vi "Engine.vi"(7 "Action":T1, 8 "error in (no error)":errorcluster, 10 "skvc in":string[](array[string]), 11 "INI Path in":path) -> (0 "error out":errorcluster, 1 "Found?":bool, 2 "skvc out":string[](array[string]), 3 "INI Path out":path)   [LabVIEW 2018, in "Cfg.lvlib"]
uses:
  Cfg.lvlib
  Action.ctl
  <vilib>/ErrorRing/Error Ring.xnode
  <vilib>/Utility/error.llb/Error Cluster From Error Code.vi
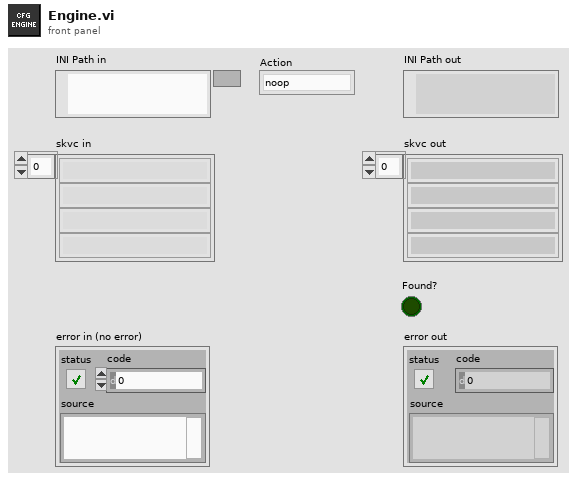
[diagram p1: front panel]
types:
  T1 = typedef "Cfg.lvlib/Action.ctl" = enum8{"noop", "new", "read_or_create", "read", "write", "remove", "keys", "sections", "remove_section", "import", "export", "get", "set", "pop", "add", "list", "list_sections", "pop_section"}
  T2 = cluster{"Paths":path[], "Files":cluster{"skvc":string[][]}[], "Modified":bool[], "LastMod":timestamp[], "PathIdx":i32, "Create":bool, "Found":bool, "skvc":string[]}
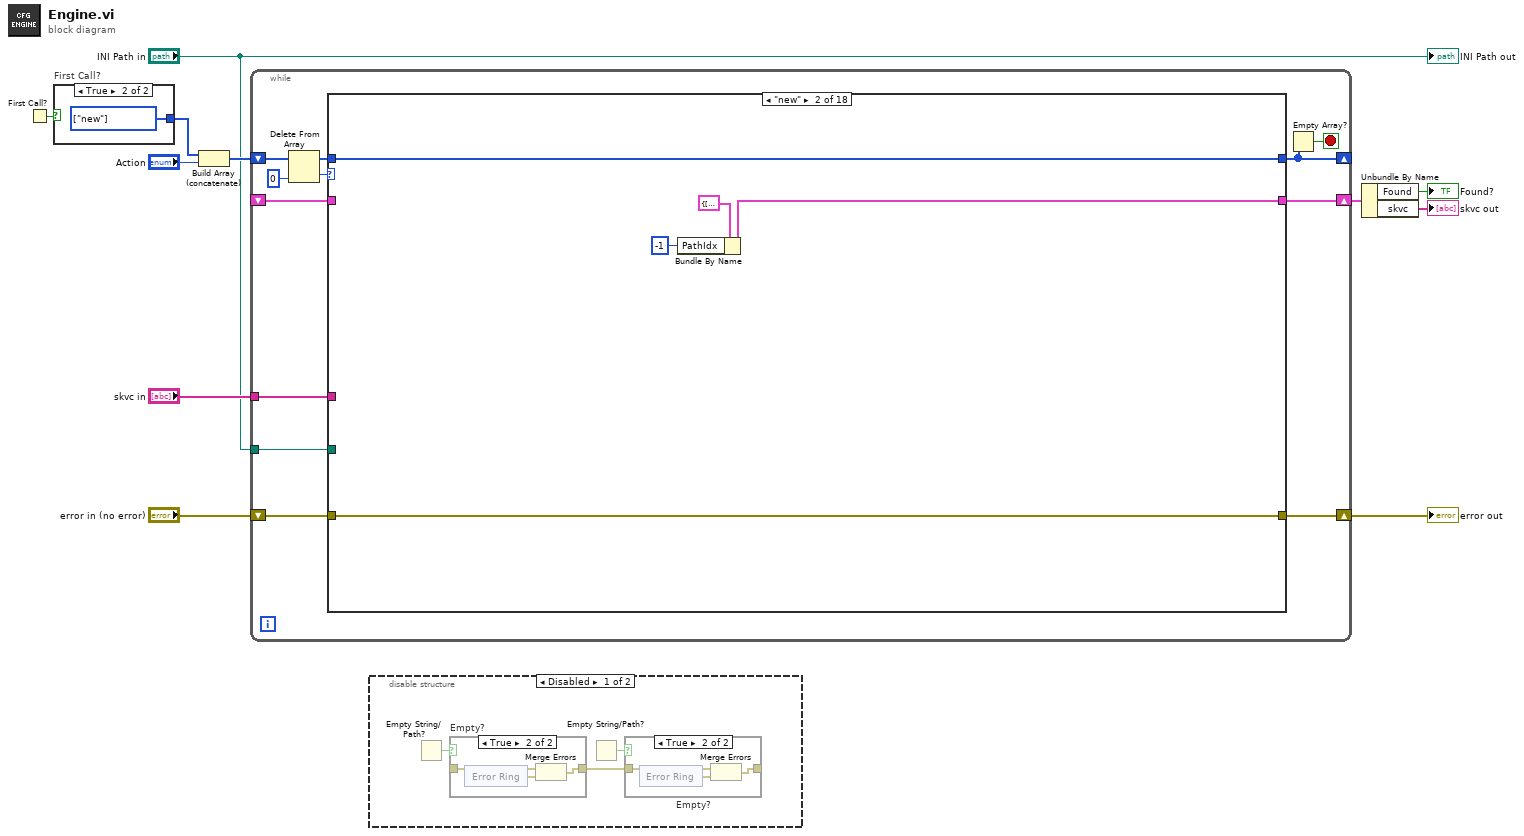
[diagram p0: block diagram]
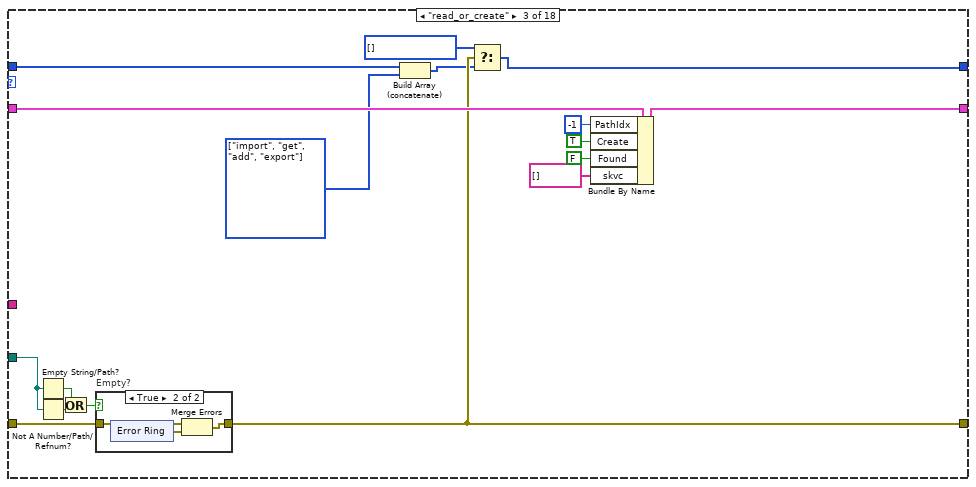
[diagram p6: hidden frame]
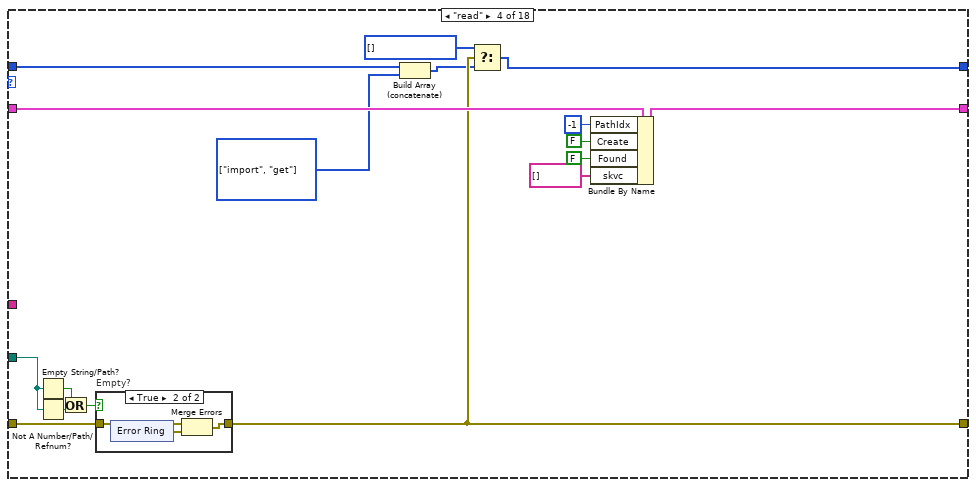
[diagram p8: hidden frame]
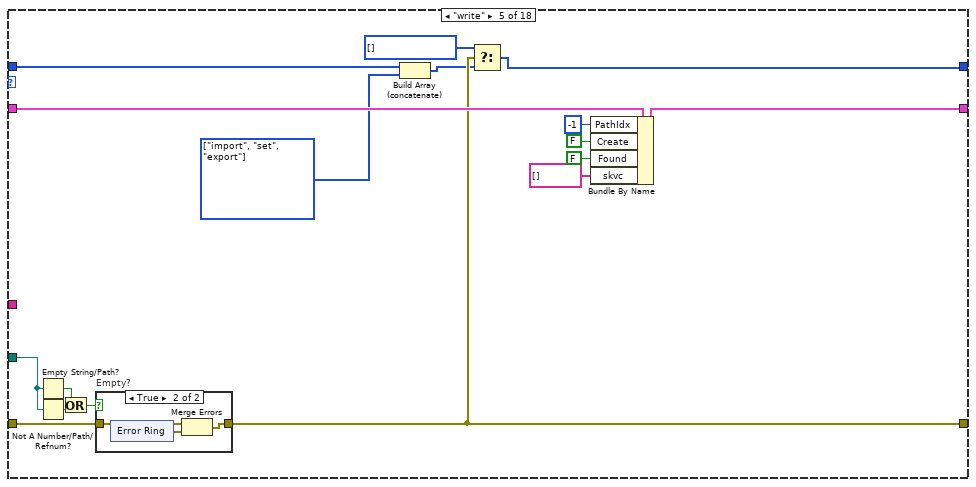
[diagram p10: hidden frame]
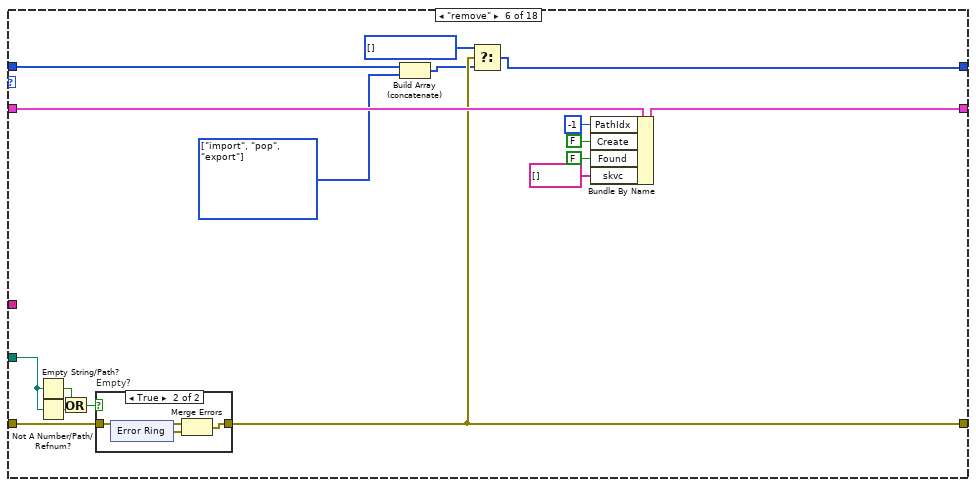
[diagram p12: hidden frame]
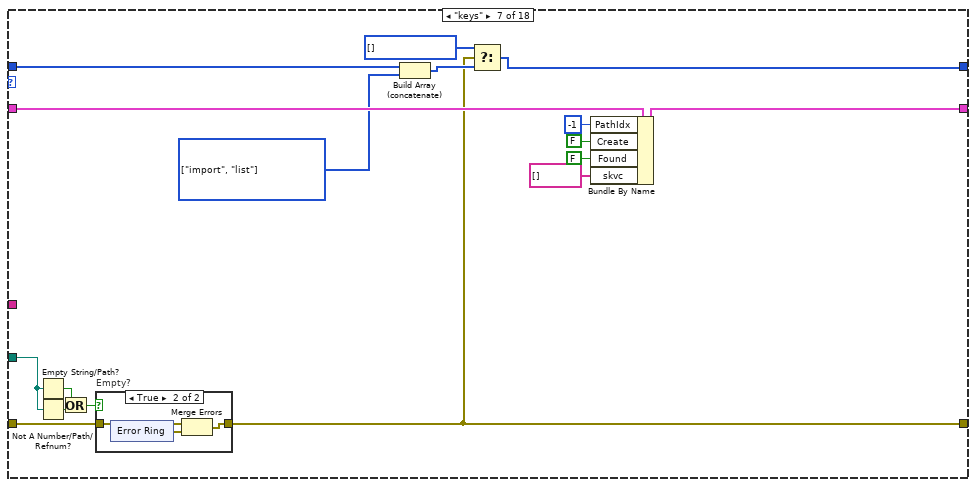
[diagram p14: hidden frame]
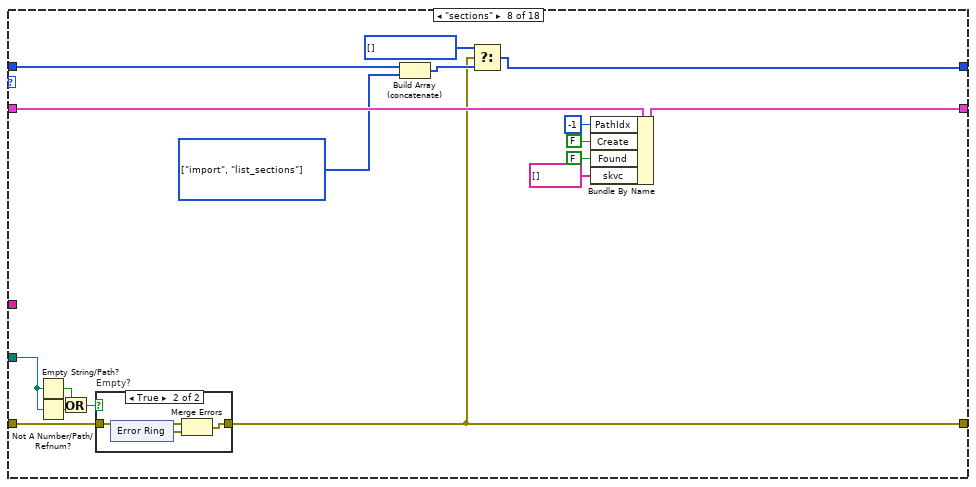
[diagram p16: hidden frame]
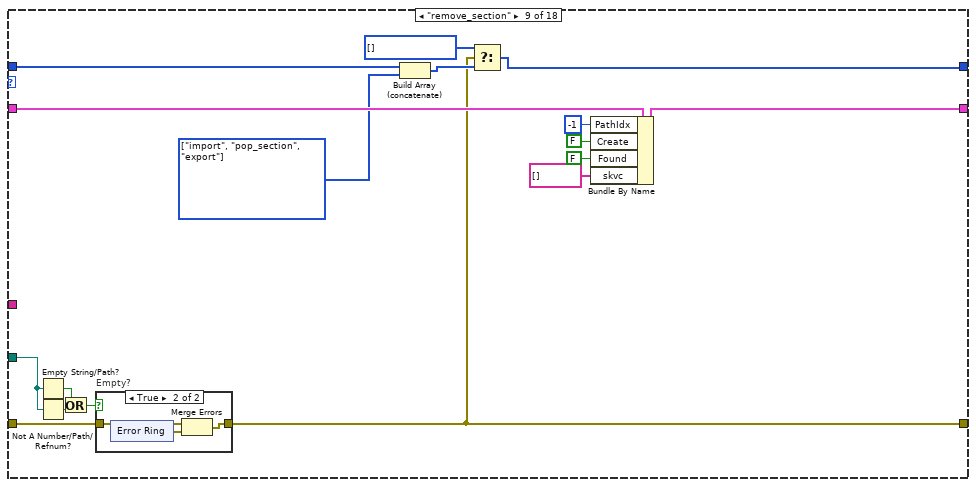
[diagram p18: hidden frame]
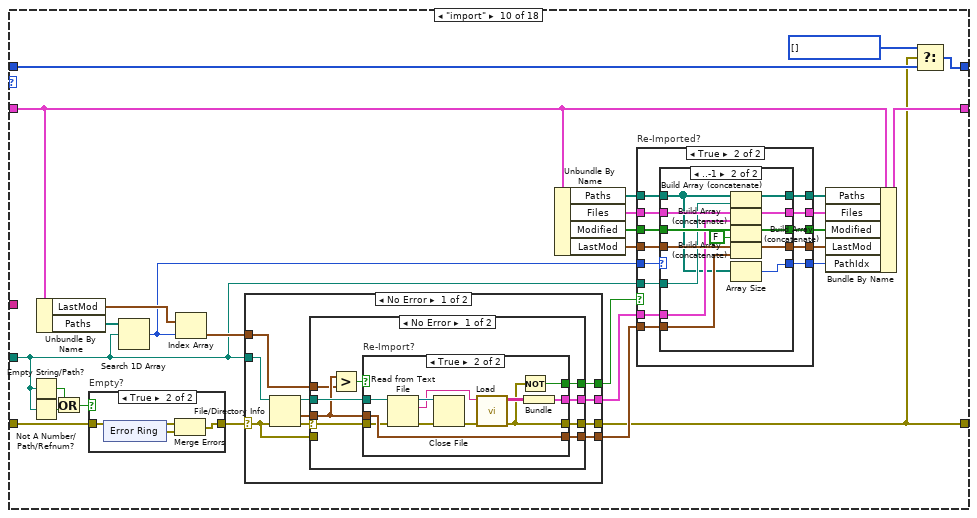
[diagram p20: hidden frame]
diagram:
  n1 = First Call?() -> (First Call?: T/F=w7:bool)
  n2 = case "First Call?" shown="True" w7 {
    tunnel: [_ w12] -> w6
    frame False {
    }
    frame True {
      w12 = T1[] [enum."new"] items=["noop", "new", "read_or_create", "read", "write", "remove", "keys", "sections", "remove_section", "import", "export", "get", "set", "pop", "add", "list", "list_sections", "pop_section"] ("appended array")
    }
  }
  n3 = Build Array (concatenate)(w6, "Action") -> (w8:T1[])
  n4 = while {
    shift-right: [w24] -> w11
    shift-left: "error in (no error)" -> [w23]
    shift-right: [w18] -> _
    shift-left: w8 -> [w22]
    shift-right: [w16] -> w3
    shift-left: _ -> [w15]
    tunnel: "INI Path in" -> [w14]
    tunnel: "skvc in" -> [w13]
    stop <- w17 stop-if-true
    n5 = Delete From Array(array=w22, index=0) -> (deleted portion=w19:T1, array with subset deleted=w21:T1[])  [unwired: 1 in]
    n6 = case shown="\"new\"" w19 {
      tunnel: [w27 w32 w41 w67 w93 w119 w137 w163 w189 w216 w339 w397 w428 w485 w529 w592 w615 w646] -> w24
      tunnel: w23 -> [w27 w32 w44 w70 w96 w122 w148 w174 w200 w241 w342 w397 w428 w485 w529 w592 w615 w646]
      tunnel: w21 -> [w26 w31 w49 w75 w101 w127 w153 w179 w205 w242 w350 w414 w431 w488 w538 w601 w622 w649]
      tunnel: [w26 w31 w42 w68 w94 w120 w146 w172 w198 w218 w350 w414 w431 w488 w538 w601 w622 w649] -> w18
      tunnel: [w25 w29 w37 w63 w89 w115 w142 w168 w194 w232 w331 w404 w429 w486 w536 w595 w616 w647] -> w16
      tunnel: w15 -> [w25 _ w48 w74 w100 w126 w152 w178 w204 w233 w336 w413 w430 w487 w537 w600 w621 w648]
      tunnel: w14 -> [_ _ w43 w69 w95 w121 w147 w173 w199 w221 w340 _ _ _ _ _ _ _]
      tunnel: w13 -> [_ _ _ _ _ _ _ _ _ _ _ w400 w426 w478 w534 w594 _ w639]
      frame "noop" {
      }
      frame "new" {
        n7 = Bundle By Name(cluster=T2 {"Paths"=[], "Files"=[], "Modified"=[], "LastMod"=[], "PathIdx"=0, "Create"=FALSE, "Found"=FALSE, "skvc"=[]} ("StateData"), "PathIdx"=-1) -> (w29:T2)
      }
      frame "read_or_create" {
        w38 = T1[] [enum."import", enum."get", enum."add", enum."export"] items=["noop", "new", "read_or_create", "read", "write", "remove", "keys", "sections", "remove_section", "import", "export", "get", "set", "pop", "add", "list", "list_sections", "pop_section"] ("element")
        w40 = T1[] [] items=["noop", "new", "read_or_create", "read", "write", "remove", "keys", "sections", "remove_section", "import", "export", "get", "set", "pop", "add", "list", "list_sections", "pop_section"] ("t")
        n8 = Empty String/Path?(string/path=w43) -> (empty?=w46:bool)
        n9 = Not A Number/Path/Refnum?(number/path/refnum=w43) -> (NaN/Path/Refnum?=w47:bool)
        n10 = Or(x=w46, y=w47) -> (x .or. y?=w45:bool)
        n11 = case "Empty?" shown="True" w45 {
          tunnel: w44 -> [w50 w53]
          tunnel: [w50 w52] -> w41
          frame False {
          }
          frame True {
            n12 = xnode "Error Ring"() -> ("error out"=w51:errorcluster)
            n13 = Merge Errors(w53, w51) -> (w52:errorcluster)
          }
        }
        n14 = Build Array (concatenate)(w49, w38) -> (w39:T1[])
        n15 = Select(t=w40, s=w41, f=w39) -> (s? t:f=w42:T1[])
        n16 = Bundle By Name(cluster=w48, "PathIdx"=-1, "Create"=TRUE, "Found"=FALSE, "skvc"=string[] []) -> (w37:T2)
      }
      frame "read" {
        w64 = T1[] [enum."import", enum."get"] items=["noop", "new", "read_or_create", "read", "write", "remove", "keys", "sections", "remove_section", "import", "export", "get", "set", "pop", "add", "list", "list_sections", "pop_section"] ("element")
        w66 = T1[] [] items=["noop", "new", "read_or_create", "read", "write", "remove", "keys", "sections", "remove_section", "import", "export", "get", "set", "pop", "add", "list", "list_sections", "pop_section"] ("t")
        n17 = Empty String/Path?(string/path=w69) -> (empty?=w72:bool)
        n18 = Not A Number/Path/Refnum?(number/path/refnum=w69) -> (NaN/Path/Refnum?=w73:bool)
        n19 = Or(x=w72, y=w73) -> (x .or. y?=w71:bool)
        n20 = case "Empty?" shown="True" w71 {
          tunnel: w70 -> [w76 w79]
          tunnel: [w76 w78] -> w67
          frame False {
          }
          frame True {
            n21 = xnode "Error Ring"() -> ("error out"=w77:errorcluster)
            n22 = Merge Errors(w79, w77) -> (w78:errorcluster)
          }
        }
        n23 = Build Array (concatenate)(w75, w64) -> (w65:T1[])
        n24 = Select(t=w66, s=w67, f=w65) -> (s? t:f=w68:T1[])
        n25 = Bundle By Name(cluster=w74, "PathIdx"=-1, "Create"=FALSE, "Found"=FALSE, "skvc"=string[] []) -> (w63:T2)
      }
      frame "write" {
        w90 = T1[] [enum."import", enum."set", enum."export"] items=["noop", "new", "read_or_create", "read", "write", "remove", "keys", "sections", "remove_section", "import", "export", "get", "set", "pop", "add", "list", "list_sections", "pop_section"] ("element")
        w92 = T1[] [] items=["noop", "new", "read_or_create", "read", "write", "remove", "keys", "sections", "remove_section", "import", "export", "get", "set", "pop", "add", "list", "list_sections", "pop_section"] ("t")
        n26 = Empty String/Path?(string/path=w95) -> (empty?=w98:bool)
        n27 = Not A Number/Path/Refnum?(number/path/refnum=w95) -> (NaN/Path/Refnum?=w99:bool)
        n28 = Or(x=w98, y=w99) -> (x .or. y?=w97:bool)
        n29 = case "Empty?" shown="True" w97 {
          tunnel: w96 -> [w102 w105]
          tunnel: [w102 w104] -> w93
          frame False {
          }
          frame True {
            n30 = xnode "Error Ring"() -> ("error out"=w103:errorcluster)
            n31 = Merge Errors(w105, w103) -> (w104:errorcluster)
          }
        }
        n32 = Build Array (concatenate)(w101, w90) -> (w91:T1[])
        n33 = Select(t=w92, s=w93, f=w91) -> (s? t:f=w94:T1[])
        n34 = Bundle By Name(cluster=w100, "PathIdx"=-1, "Create"=FALSE, "Found"=FALSE, "skvc"=string[] []) -> (w89:T2)
      }
      frame "remove" {
        w116 = T1[] [enum."import", enum."pop", enum."export"] items=["noop", "new", "read_or_create", "read", "write", "remove", "keys", "sections", "remove_section", "import", "export", "get", "set", "pop", "add", "list", "list_sections", "pop_section"] ("element")
        w118 = T1[] [] items=["noop", "new", "read_or_create", "read", "write", "remove", "keys", "sections", "remove_section", "import", "export", "get", "set", "pop", "add", "list", "list_sections", "pop_section"] ("t")
        n35 = Empty String/Path?(string/path=w121) -> (empty?=w124:bool)
        n36 = Not A Number/Path/Refnum?(number/path/refnum=w121) -> (NaN/Path/Refnum?=w125:bool)
        n37 = Or(x=w124, y=w125) -> (x .or. y?=w123:bool)
        n38 = case "Empty?" shown="True" w123 {
          tunnel: w122 -> [w128 w131]
          tunnel: [w128 w130] -> w119
          frame False {
          }
          frame True {
            n39 = xnode "Error Ring"() -> ("error out"=w129:errorcluster)
            n40 = Merge Errors(w131, w129) -> (w130:errorcluster)
          }
        }
        n41 = Build Array (concatenate)(w127, w116) -> (w117:T1[])
        n42 = Select(t=w118, s=w119, f=w117) -> (s? t:f=w120:T1[])
        n43 = Bundle By Name(cluster=w126, "PathIdx"=-1, "Create"=FALSE, "Found"=FALSE, "skvc"=string[] []) -> (w115:T2)
      }
      frame "keys" {
        w143 = T1[] [enum."import", enum."list"] items=["noop", "new", "read_or_create", "read", "write", "remove", "keys", "sections", "remove_section", "import", "export", "get", "set", "pop", "add", "list", "list_sections", "pop_section"] ("element")
        w145 = T1[] [] items=["noop", "new", "read_or_create", "read", "write", "remove", "keys", "sections", "remove_section", "import", "export", "get", "set", "pop", "add", "list", "list_sections", "pop_section"] ("t")
        n44 = Empty String/Path?(string/path=w147) -> (empty?=w150:bool)
        n45 = Not A Number/Path/Refnum?(number/path/refnum=w147) -> (NaN/Path/Refnum?=w151:bool)
        n46 = Or(x=w150, y=w151) -> (x .or. y?=w149:bool)
        n47 = case "Empty?" shown="True" w149 {
          tunnel: w148 -> [w154 w157]
          tunnel: [w154 w156] -> w137
          frame False {
          }
          frame True {
            n48 = xnode "Error Ring"() -> ("error out"=w155:errorcluster)
            n49 = Merge Errors(w157, w155) -> (w156:errorcluster)
          }
        }
        n50 = Build Array (concatenate)(w153, w143) -> (w144:T1[])
        n51 = Select(t=w145, s=w137, f=w144) -> (s? t:f=w146:T1[])
        n52 = Bundle By Name(cluster=w152, "PathIdx"=-1, "Create"=FALSE, "Found"=FALSE, "skvc"=string[] []) -> (w142:T2)
      }
      frame "sections" {
        w169 = T1[] [enum."import", enum."list_sections"] items=["noop", "new", "read_or_create", "read", "write", "remove", "keys", "sections", "remove_section", "import", "export", "get", "set", "pop", "add", "list", "list_sections", "pop_section"] ("element")
        w171 = T1[] [] items=["noop", "new", "read_or_create", "read", "write", "remove", "keys", "sections", "remove_section", "import", "export", "get", "set", "pop", "add", "list", "list_sections", "pop_section"] ("t")
        n53 = Empty String/Path?(string/path=w173) -> (empty?=w176:bool)
        n54 = Not A Number/Path/Refnum?(number/path/refnum=w173) -> (NaN/Path/Refnum?=w177:bool)
        n55 = Or(x=w176, y=w177) -> (x .or. y?=w175:bool)
        n56 = case "Empty?" shown="True" w175 {
          tunnel: w174 -> [w180 w183]
          tunnel: [w180 w182] -> w163
          frame False {
          }
          frame True {
            n57 = xnode "Error Ring"() -> ("error out"=w181:errorcluster)
            n58 = Merge Errors(w183, w181) -> (w182:errorcluster)
          }
        }
        n59 = Build Array (concatenate)(w179, w169) -> (w170:T1[])
        n60 = Select(t=w171, s=w163, f=w170) -> (s? t:f=w172:T1[])
        n61 = Bundle By Name(cluster=w178, "PathIdx"=-1, "Create"=FALSE, "Found"=FALSE, "skvc"=string[] []) -> (w168:T2)
      }
      frame "remove_section" {
        w195 = T1[] [enum."import", enum."pop_section", enum."export"] items=["noop", "new", "read_or_create", "read", "write", "remove", "keys", "sections", "remove_section", "import", "export", "get", "set", "pop", "add", "list", "list_sections", "pop_section"] ("element")
        w197 = T1[] [] items=["noop", "new", "read_or_create", "read", "write", "remove", "keys", "sections", "remove_section", "import", "export", "get", "set", "pop", "add", "list", "list_sections", "pop_section"] ("t")
        n62 = Empty String/Path?(string/path=w199) -> (empty?=w202:bool)
        n63 = Not A Number/Path/Refnum?(number/path/refnum=w199) -> (NaN/Path/Refnum?=w203:bool)
        n64 = Or(x=w202, y=w203) -> (x .or. y?=w201:bool)
        n65 = case "Empty?" shown="True" w201 {
          tunnel: w200 -> [w206 w209]
          tunnel: [w206 w208] -> w189
          frame False {
          }
          frame True {
            n66 = xnode "Error Ring"() -> ("error out"=w207:errorcluster)
            n67 = Merge Errors(w209, w207) -> (w208:errorcluster)
          }
        }
        n68 = Build Array (concatenate)(w205, w195) -> (w196:T1[])
        n69 = Select(t=w197, s=w189, f=w196) -> (s? t:f=w198:T1[])
        n70 = Bundle By Name(cluster=w204, "PathIdx"=-1, "Create"=FALSE, "Found"=FALSE, "skvc"=string[] []) -> (w194:T2)
      }
      frame "import" {
        w217 = T1[] [] items=["noop", "new", "read_or_create", "read", "write", "remove", "keys", "sections", "remove_section", "import", "export", "get", "set", "pop", "add", "list", "list_sections", "pop_section"] ("t")
        n71 = Empty String/Path?(string/path=w221) -> (empty?=w237:bool)
        n72 = Not A Number/Path/Refnum?(number/path/refnum=w221) -> (NaN/Path/Refnum?=w238:bool)
        n73 = Unbundle By Name(w233) -> ("LastMod"=w240:timestamp[], "Paths"=w234:path[])
        n74 = Or(x=w237, y=w238) -> (x .or. y?=w236:bool)
        n75 = case "Empty?" shown="True" w236 {
          tunnel: w241 -> [w319 w322]
          tunnel: [w319 w321] -> w235
          frame False {
          }
          frame True {
            n76 = xnode "Error Ring"() -> ("error out"=w320:errorcluster)
            n77 = Merge Errors(w322, w320) -> (w321:errorcluster)
          }
        }
        n78 = Search 1D Array(1D array=w234, element=w221) -> (index of element=w219:i32)  [unwired: 1 in]
        n79 = Index Array(array=w240, index=w219) -> (element=w239:timestamp)
        n80 = case shown="No Error" w235 {
          selector: w235 -> [w288 w318]
          tunnel: [w294 w318] -> w216
          tunnel: w239 -> [w290 _]
          tunnel: w221 -> [w289 _]
          tunnel: [w287 _] -> w222
          tunnel: [w286 _] -> w220
          tunnel: [w285 _] -> w223
          frame No Error {
            n81 = File/Directory Info(path=w289, error in=w288) -> (path out=w292:path, last mod=w291:timestamp, error out=w293:errorcluster)  [unwired: 4 out]
            n82 = case shown="No Error" w293 {
              selector: w293 -> [w296 _]
              tunnel: [w297 w317] -> w294
              tunnel: w292 -> [w303 _]
              tunnel: w291 -> [w301 _]
              tunnel: w290 -> [w298 _]
              tunnel: w288 -> [_ w317]
              tunnel: [w300 _] -> w287
              tunnel: [w299 _] -> w286
              tunnel: [w295 TRUE] -> w285
              frame No Error {
                n83 = Greater?(x=w301, y=w298) -> (0:w302:bool)
                n84 = case "Re-Import?" shown="True" w302 {
                  tunnel: w303 -> [_ w315]
                  tunnel: w301 -> [_ w309]
                  tunnel: [_ w305] -> w300
                  tunnel: [_ w309] -> w299
                  tunnel: [w304 w307] -> w297
                  tunnel: w296 -> [w304 w308]
                  tunnel: [_ w306] -> w295
                  frame False {
                  }
                  frame True {
                    n85 = Read from Text File(file (use dialog)=w315, error in=w308) -> (refnum out=w313:refnum<file>, text=w311:string, error out=w314:errorcluster)  [unwired: 2 in, 1 out]
                    n86 = Close File(refnum=w313, error in=w314) -> (error out=w312:errorcluster)  [unwired: 1 out]
                    n87 = call "Load.vi"("error in (no error)"=w312, "Text"=w311) -> ("error out"=w307:errorcluster, "skvc"=w310:string[][])  [unwired: 8 in]
                    n88 = Not(x=w307) -> (.not. x?=w306:bool)
                    n89 = Bundle("skvc"=w310) -> (w305:cluster{"skvc":string[][]})  [unwired: 1 in]
                  }
                }
              }
              frame Error {
                # "File does not exist"
              }
            }
          }
          frame Error {
          }
        }
        n90 = Unbundle By Name(w233) -> ("Paths"=w231:path[], "Files"=w230:cluster{"skvc":string[][]}[], "Modified"=w229:bool[], "LastMod"=w228:timestamp[])
        n91 = case "Re-Imported?" shown="True" w223 {
          tunnel: w231 -> [w247 w260]
          tunnel: w230 -> [w246 w259]
          tunnel: w229 -> [w245 w258]
          tunnel: w228 -> [w244 w257]
          tunnel: [w244 w256] -> w227
          tunnel: [w245 w255] -> w226
          tunnel: [w246 w254] -> w225
          tunnel: [w247 w253] -> w224
          tunnel: w222 -> [_ w252]
          tunnel: w221 -> [_ w251]
          tunnel: w220 -> [_ w250]
          tunnel: w219 -> [w243 w249]
          tunnel: [w243 w248] -> w215
          frame False {
          }
          frame True {
            n92 = case shown="..-1" w249 {
              selector: w249 -> [w262 _]
              tunnel: w260 -> [w271 w273]
              tunnel: w259 -> [w270 w284]
              tunnel: w258 -> [w264 w283]
              tunnel: w257 -> [w266 w282]
              tunnel: [w265 w281] -> w256
              tunnel: [w263 w280] -> w255
              tunnel: [w269 w279] -> w254
              tunnel: [w271 w278] -> w253
              tunnel: w252 -> [w268 w277]
              tunnel: w251 -> [_ w276]
              tunnel: w250 -> [w267 w274]
              tunnel: [w262 w272] -> w248
              frame 0.. {
                n93 = Replace Array Subset(array=w270, new element=w268, index=w262) -> (w269:cluster{"skvc":string[][]}[])
                n94 = Replace Array Subset(array=w264, new element=FALSE ("new element/subarray"), index=w262) -> (w263:bool[])
                n95 = Replace Array Subset(array=w266, new element=w267, index=w262) -> (w265:timestamp[])
              }
              frame ..-1 {
                n96 = Build Array (concatenate)(w273, w276) -> (w278:path[])
                n97 = Build Array (concatenate)(w284, w277) -> (w279:cluster{"skvc":string[][]}[])
                n98 = Build Array (concatenate)(w283, FALSE ("Boolean")) -> (w280:bool[])
                n99 = Build Array (concatenate)(w282, w274) -> (w281:timestamp[])
                n100 = Array Size(array=w273) -> (size(s)=w272:i32)
              }
            }
          }
        }
        n101 = Bundle By Name(cluster=w233, "Paths"=w224, "Files"=w225, "Modified"=w226, "LastMod"=w227, "PathIdx"=w215) -> (w232:T2)
        n102 = Select(t=w217, s=w216, f=w242) -> (s? t:f=w218:T1[])
      }
      frame "export" {
        n103 = Empty String/Path?(string/path=w340) -> (empty?=w345:bool)
        n104 = Not A Number/Path/Refnum?(number/path/refnum=w340) -> (NaN/Path/Refnum?=w346:bool)
        n105 = Unbundle By Name(w336) -> ("Files"=w347:cluster{"skvc":string[][]}[], "Modified"=w348:bool[], "Paths"=w349:path[])
        n106 = Or(x=w345, y=w346) -> (x .or. y?=w344:bool)
        n107 = case "Empty?" shown="True" w344 {
          tunnel: w342 -> [w387 w390]
          tunnel: [w387 w389] -> w343
          frame False {
          }
          frame True {
            n108 = xnode "Error Ring"() -> ("error out"=w388:errorcluster)
            n109 = Merge Errors(w390, w388) -> (w389:errorcluster)
          }
        }
        n110 = Search 1D Array(1D array=w349, element=w340) -> (index of element=w332:i32)  [unwired: 1 in]
        n111 = Index Array(array=w347, index=w332) -> (element=w341:cluster{"skvc":string[][]})
        n112 = Index Array(array=w348, index=w332) -> (element=w338:bool)
        n113 = Unbundle By Name(w341) -> ("skvc"=w337:string[][])
        n114 = case "Modified?" shown="True" w338 {
          tunnel: w343 -> [w360 w366]
          tunnel: w340 -> [_ w365]
          tunnel: [w360 w364] -> w339
          tunnel: w337 -> [_ w362]
          tunnel: [_ w363] -> w334
          tunnel: [_ w361] -> w328
          frame False {
          }
          frame True {
            n115 = case shown="No Error" w366 {
              selector: w366 -> [w382 w386]
              tunnel: w365 -> [w377 _]
              tunnel: [w372 w386] -> w364
              tunnel: [w373 _] -> w363
              tunnel: w362 -> [w367 _]
              tunnel: [w371 _] -> w361
              frame No Error {
                n116 = Strip Path(path=w377) -> (stripped path=w380:path)  [unwired: 1 out]
                n117 = File/Directory Info(path=w380, error in=w382) -> (path out=w379:path, error out=w381:errorcluster)  [unwired: 5 out]
                n118 = case shown="Error .." w381 {
                  selector: w381 -> [w383 _]
                  tunnel: [w383 w385] -> w370
                  tunnel: w379 -> [_ w384]
                  frame No Error {
                  }
                  frame Error {
                    n119 = Create Folder(path (use dialog)=w384) -> (error out=w385:errorcluster)  [unwired: 2 in, 2 out]
                  }
                }
                n120 = call "Dump.vi"("error in (no error)"=w370, "skvc"=w367) -> ("error out"=w369:errorcluster, "Text"=w368:string)  [unwired: 8 in]
                n121 = Write to Text File(file (use dialog)=w377, text=w368, error in=w369) -> (refnum out=w375:refnum<file>, error out=w378:errorcluster)  [unwired: 1 in, 1 out]
                n122 = Close File(refnum=w375, error in=w378) -> (path=w374:path, error out=w376:errorcluster)
                n123 = File/Directory Info(path=w374, error in=w376) -> (last mod=w373:timestamp, error out=w372:errorcluster)  [unwired: 5 out]
                n124 = Not(x=w372) -> (.not. x?=w371:bool)
              }
              frame Error {
              }
            }
          }
        }
        n125 = Unbundle By Name(w336) -> ("Modified"=w333:bool[], "LastMod"=w335:timestamp[])
        n126 = case "Written?" shown="True" w328 {
          tunnel: w335 -> [w351 w359]
          tunnel: w334 -> [_ w358]
          tunnel: w333 -> [w352 w357]
          tunnel: w332 -> [_ w355]
          tunnel: [w352 w354] -> w330
          tunnel: [w351 w353] -> w329
          frame False {
          }
          frame True {
            n127 = Replace Array Subset(array=w357, new element=FALSE ("new element/subarray"), index=w355) -> (w354:bool[])
            n128 = Replace Array Subset(array=w359, new element=w358, index=w355) -> (w353:timestamp[])
          }
        }
        n129 = Bundle By Name(cluster=w336, "Modified"=w330, "LastMod"=w329) -> (w331:T2)
      }
      frame "get" {
        n130 = Unbundle By Name(w413) -> ("Files"=w412:cluster{"skvc":string[][]}[], "PathIdx"=w411:i32)
        n131 = Index Array(array=w412, index=w411) -> (element=w410:cluster{"skvc":string[][]})
        n132 = Unbundle By Name(w410) -> ("skvc"=w405:string[][])
        n133 = for {
          tunnel: w405 -> [w420] mode=indexing
          tunnel: [w417] -> w409 mode=indexing
          n134 = Index Array(array=w420) -> (element #1=w419:string, element #2=w418:string)  [unwired: 2 in]
          n135 = To Upper Case(1:w419) -> (0:w415:string)
          n136 = To Upper Case(1:w418) -> (0:w416:string)
          n137 = Bundle(w415, w416) -> (w417:cluster{string, string})  [unwired: 1 in]
        }
        n138 = Index Array(array=w400) -> (element #1=w399:string, element #2=w398:string)  [unwired: 2 in]
        n139 = To Upper Case(1:w399) -> (0:w408:string)
        n140 = To Upper Case(1:w398) -> (0:w407:string)
        n141 = Bundle(w408, w407) -> (w406:cluster{string, string})  [unwired: 1 in]
        n142 = Search 1D Array(1D array=w409, element=w406) -> (index of element=w403:i32)  [unwired: 1 in]
        n143 = Greater Or Equal To 0?(x=w403) -> (x >= 0?=w396:bool)
        n144 = Index Array(array=w405, index (row)=w403) -> (element=w402:string[])  [unwired: 1 in]
        n145 = Select(t=w402, s=w396, f=w400) -> (s? t:f=w401:string[])
        n146 = Bundle By Name(cluster=w413, "skvc"=w401, "Found"=w396) -> (w404:T2)
      }
      frame "set" {
        n147 = Unbundle By Name(w430) -> ("Modified"=w423:bool[], "Files"=w427:cluster{"skvc":string[][]}[], "PathIdx"=w424:i32)
        n148 = in-place {
          in-place-border: w426 -> [w437]
          in-place-border: [w432] -> w421
          n149 = in-place-array #1(w423, w424) -> (w434:bool)
          n150 = in-place-array #2(w427, w424) -> (w436:cluster{"skvc":string[][]})
          n151 = in-place {
            in-place-border: w437 -> [w441]
            in-place-border: w434 -> [w440]
            in-place-border: [w439] -> w433
            in-place-border: [w438] -> w432
            n152 = in-place-cluster #3(w436) -> ("skvc"=w443:string[][])
            n153 = for {
              tunnel: w443 -> [w476] mode=indexing
              tunnel: [w473] -> w450 mode=indexing
              n154 = Index Array(array=w476) -> (element #1=w475:string, element #2=w474:string)  [unwired: 2 in]
              n155 = To Upper Case(1:w475) -> (0:w471:string)
              n156 = To Upper Case(1:w474) -> (0:w472:string)
              n157 = Bundle(w471, w472) -> (w473:cluster{string, string})  [unwired: 1 in]
            }
            n158 = Index Array(array=w441) -> (element #1=w446:string, element #2=w445:string)  [unwired: 2 in]
            n159 = To Upper Case(1:w446) -> (0:w449:string)
            n160 = To Upper Case(1:w445) -> (0:w448:string)
            n161 = Bundle(w449, w448) -> (w447:cluster{string, string})  [unwired: 1 in]
            n162 = Search 1D Array(1D array=w450, element=w447) -> (index of element=w444:i32)  [unwired: 1 in]
            n163 = case shown="0.." w444 {
              selector: w444 -> [w455 _]
              tunnel: w443 -> [w458 w470]
              tunnel: [w456 w469] -> w442
              tunnel: w441 -> [w454 w468]
              tunnel: w440 -> [w453 _]
              tunnel: [w452 w467] -> w439
              tunnel: [w451 w466] -> w438
              frame 0.. {
                w451 = TRUE  # Found?
                n164 = in-place {
                  in-place-border: w454 -> [w465]
                  in-place-border: w453 -> [w462]
                  in-place-border: [w460] -> w452
                  n165 = in-place-array #4(w458, w455, 2) -> (w463:string)
                  n166 = Index Array(array=w465, index=2) -> (element=w459:string)
                  n167 = Not Equal?(x=w463, y=w459) -> (x != y?=w461:bool)
                  n168 = Or(x=w462, y=w461) -> (x .or. y?=w460:bool)
                  n169 = in-place-array #4(w459) -> (w456:string[][])  [unwired: 2 out]
                }
              }
              frame ..-1 {
                w466 = FALSE  # Found?
                w467 = TRUE  # Modified?
                n170 = Build Array (concatenate)(w470, w468) -> (w469:string[][])
              }
            }
            n171 = in-place-cluster #3("skvc"=w442) -> (w435:cluster{"skvc":string[][]})
          }
          n172 = in-place-array #1(w433) -> (w422:bool[])  [unwired: 1 out]
          n173 = in-place-array #2(w435) -> (w425:cluster{"skvc":string[][]}[])  [unwired: 1 out]
        }
        n174 = Bundle By Name(cluster=w430, "Modified"=w422, "Files"=w425, "Found"=w421, "skvc"=w426) -> (w429:T2)
      }
      frame "pop" {
        n175 = Unbundle By Name(w487) -> ("Modified"=w481:bool[], "Files"=w484:cluster{"skvc":string[][]}[], "PathIdx"=w482:i32)
        n176 = in-place {
          in-place-border: w478 -> [w495]
          in-place-border: [w490] -> w479
          in-place-border: [w489] -> w477
          n177 = in-place-array #5(w481, w482) -> (w492:bool)
          n178 = in-place-array #6(w484, w482) -> (w494:cluster{"skvc":string[][]})
          n179 = in-place {
            in-place-border: w495 -> [w497]
            in-place-border: w492 -> [w501]
            in-place-border: [w500] -> w491
            in-place-border: [w499] -> w490
            in-place-border: [w496] -> w489
            n180 = in-place-cluster #7(w494) -> ("skvc"=w502:string[][])
            n181 = for {
              tunnel: w502 -> [w525] mode=indexing
              tunnel: [w522] -> w509 mode=indexing
              n182 = Index Array(array=w525) -> (element #1=w524:string, element #2=w523:string)  [unwired: 2 in]
              n183 = To Upper Case(1:w524) -> (0:w520:string)
              n184 = To Upper Case(1:w523) -> (0:w521:string)
              n185 = Bundle(w520, w521) -> (w522:cluster{string, string})  [unwired: 1 in]
            }
            n186 = Index Array(array=w497) -> (element #1=w505:string, element #2=w504:string)  [unwired: 2 in]
            n187 = To Upper Case(1:w505) -> (0:w508:string)
            n188 = To Upper Case(1:w504) -> (0:w507:string)
            n189 = Bundle(w508, w507) -> (w506:cluster{string, string})  [unwired: 1 in]
            n190 = Search 1D Array(1D array=w509, element=w506) -> (index of element=w503:i32)  [unwired: 1 in]
            n191 = case shown="0.." w503 {
              selector: w503 -> [w513 _]
              tunnel: w502 -> [w514 w518]
              tunnel: w501 -> [_ w517]
              tunnel: [w511 w517] -> w500
              tunnel: [w515 w519] -> w499
              tunnel: [w512 w518] -> w498
              tunnel: w497 -> [_ w516]
              tunnel: [w510 w516] -> w496
              frame 0.. {
                w511 = TRUE  # Modified?
                w515 = TRUE  # Found?
                n192 = Delete From Array(array=w514, index (row)=w513) -> (deleted portion=w510:string[], array with subset deleted=w512:string[][])  [unwired: 2 in]
              }
              frame ..-1 {
                w519 = FALSE  # Found?
              }
            }
            n193 = in-place-cluster #7("skvc"=w498) -> (w493:cluster{"skvc":string[][]})
          }
          n194 = in-place-array #5(w491) -> (w480:bool[])  [unwired: 1 out]
          n195 = in-place-array #6(w493) -> (w483:cluster{"skvc":string[][]}[])  [unwired: 1 out]
        }
        n196 = Bundle By Name(cluster=w487, "Modified"=w480, "Files"=w483, "Found"=w479, "skvc"=w477) -> (w486:T2)
      }
      frame "add" {
        n197 = Unbundle By Name(w537) -> ("Create"=w528:bool, "Found"=w527:bool, "Modified"=w531:bool[], "Files"=w535:cluster{"skvc":string[][]}[], "PathIdx"=w532:i32)
        n198 = Compound Arithmetic op=AND(w528, invert w527) -> (w526:bool)
        n199 = case "Create Key?" shown="True" w526 {
          tunnel: w535 -> [w539 w546]
          tunnel: w534 -> [_ w545]
          tunnel: [w539 w544] -> w533
          tunnel: w532 -> [_ w543]
          tunnel: w531 -> [w540 w542]
          tunnel: [w540 w541] -> w530
          frame False {
          }
          frame True {
            n200 = in-place {
              in-place-border: w545 -> [w551]
              n201 = in-place-array #8(w542, w543) -> (w548:bool)
              n202 = in-place-array #9(w546, w543) -> (w550:cluster{"skvc":string[][]})
              n203 = in-place {
                in-place-border: w551 -> [w554]
                in-place-border: w548 -> [w553]
                in-place-border: [w552] -> w547
                n204 = in-place-cluster #10(w550) -> ("skvc"=w556:string[][])
                n205 = for {
                  tunnel: w556 -> [w587] mode=indexing
                  tunnel: [w584] -> w563 mode=indexing
                  n206 = Index Array(array=w587) -> (element #1=w586:string, element #2=w585:string)  [unwired: 2 in]
                  n207 = To Upper Case(1:w586) -> (0:w582:string)
                  n208 = To Upper Case(1:w585) -> (0:w583:string)
                  n209 = Bundle(w582, w583) -> (w584:cluster{string, string})  [unwired: 1 in]
                }
                n210 = Index Array(array=w554) -> (element #1=w559:string, element #2=w558:string)  [unwired: 2 in]
                n211 = To Upper Case(1:w559) -> (0:w562:string)
                n212 = To Upper Case(1:w558) -> (0:w561:string)
                n213 = Bundle(w562, w561) -> (w560:cluster{string, string})  [unwired: 1 in]
                n214 = Search 1D Array(1D array=w563, element=w560) -> (index of element=w557:i32)  [unwired: 1 in]
                n215 = case shown="0.." w557 {
                  selector: w557 -> [w567 _]
                  tunnel: w556 -> [w570 w581]
                  tunnel: [w568 w580] -> w555
                  tunnel: w554 -> [w566 w579]
                  tunnel: w553 -> [w565 _]
                  tunnel: [w564 w578] -> w552
                  frame 0.. {
                    n216 = in-place {
                      in-place-border: w566 -> [w577]
                      in-place-border: w565 -> [w574]
                      in-place-border: [w572] -> w564
                      n217 = in-place-array #11(w570, w567, 2) -> (w575:string)
                      n218 = Index Array(array=w577, index=2) -> (element=w571:string)
                      n219 = Not Equal?(x=w575, y=w571) -> (x != y?=w573:bool)
                      n220 = Or(x=w574, y=w573) -> (x .or. y?=w572:bool)
                      n221 = in-place-array #11(w571) -> (w568:string[][])  [unwired: 2 out]
                    }
                  }
                  frame ..-1 {
                    w578 = TRUE  # Modified?
                    n222 = Build Array (concatenate)(w581, w579) -> (w580:string[][])
                  }
                }
                n223 = in-place-cluster #10("skvc"=w555) -> (w549:cluster{"skvc":string[][]})
              }
              n224 = in-place-array #8(w547) -> (w541:bool[])  [unwired: 1 out]
              n225 = in-place-array #9(w549) -> (w544:cluster{"skvc":string[][]}[])  [unwired: 1 out]
            }
          }
        }
        n226 = Bundle By Name(cluster=w537, "Modified"=w530, "Files"=w533) -> (w536:T2)
      }
      frame "list" {
        n227 = Unbundle By Name(w600) -> ("Files"=w599:cluster{"skvc":string[][]}[], "PathIdx"=w598:i32)
        n228 = Index Array(array=w594) -> (element=w593:string)  [unwired: 1 in]
        n229 = Index Array(array=w599, index=w598) -> (element=w597:cluster{"skvc":string[][]})
        n230 = To Upper Case(1:w593) -> (0:w591:string)
        n231 = Unbundle By Name(w597) -> ("skvc"=w596:string[][])
        n232 = for {
          tunnel: w596 -> [w611] mode=indexing
          tunnel: [w607] -> w590 mode=indexing if=w605
          tunnel: w591 -> [w608]
          shift-right: [w603] -> w588
          shift-left: FALSE -> [w602]
          n233 = Index Array(array=w611) -> (element #1=w610:string, element #2=w607:string)  [unwired: 2 in]
          n234 = To Upper Case(1:w610) -> (0:w609:string)
          n235 = Equal?(x=w609, y=w608) -> (x = y?=w604:bool)
          n236 = Empty String/Path?(string/path=w607) -> (empty?=w606:bool)
          n237 = Or(x=w604, y=w602) -> (x .or. y?=w603:bool)
          n238 = Compound Arithmetic op=AND(invert w606, w604) -> (w605:bool)
        }
        n239 = Bundle By Name(cluster=w600, "skvc"=w590, "Found"=w588) -> (w595:T2)
      }
      frame "list_sections" {
        n240 = Unbundle By Name(w621) -> ("Files"=w620:cluster{"skvc":string[][]}[], "PathIdx"=w619:i32)
        n241 = Index Array(array=w620, index=w619) -> (element=w618:cluster{"skvc":string[][]})
        n242 = Unbundle By Name(w618) -> ("skvc"=w617:string[][])
        n243 = for {
          tunnel: w617 -> [w626] mode=indexing
          shift-right: [w625] -> w612
          shift-left: string[] [] -> [w624]
          n244 = Index Array(array=w626) -> (element=w623:string)  [unwired: 1 in]
          n245 = case shown="Default" w623 {
            selector: w623 -> [_ w628]
            tunnel: [w627 w630] -> w625
            tunnel: w624 -> [w627 w629]
            frame "" {
            }
            frame Default {
              n246 = To Upper Case(1:w629) -> (0:w633:string[])
              n247 = To Upper Case(1:w628) -> (0:w632:string)
              n248 = Search 1D Array(1D array=w633, element=w632) -> (index of element=w631:i32)  [unwired: 1 in]
              n249 = case shown="..-1" w631 {
                tunnel: [w634 w636] -> w630
                tunnel: w629 -> [w634 w637]
                tunnel: w628 -> [_ w635]
                frame 0.. {
                }
                frame ..-1 {
                  n250 = Build Array (concatenate)(w637, w635) -> (w636:string[])
                }
              }
            }
          }
        }
        n251 = Bundle By Name(cluster=w621, "skvc"=w612, "Found"=FALSE) -> (w616:T2)
      }
      frame "pop_section" {
        n252 = Unbundle By Name(w648) -> ("Modified"=w642:bool[], "Files"=w645:cluster{"skvc":string[][]}[], "PathIdx"=w643:i32)
        n253 = in-place {
          in-place-border: w639 -> [w655]
          in-place-border: [w650] -> w640
          n254 = in-place-array #12(w642, w643) -> (w652:bool)
          n255 = in-place-array #13(w645, w643) -> (w654:cluster{"skvc":string[][]})
          n256 = in-place {
            in-place-border: w655 -> [w662]
            in-place-border: w652 -> [w663]
            in-place-border: [w657] -> w651
            in-place-border: [w656] -> w650
            n257 = in-place-cluster #14(w654) -> ("skvc"=w660:string[][])
            n258 = Index Array(array=w662) -> (element=w664:string)  [unwired: 1 in]
            n259 = To Upper Case(1:w664) -> (0:w661:string)
            n260 = for {
              tunnel: w660 -> [w668] mode=indexing
              tunnel: w661 -> [w669]
              tunnel: [w668] -> w659 mode=indexing if=w667
              shift-right: [w665] -> w656
              shift-left: FALSE -> [w666]
              n261 = Index Array(array=w668) -> (element=w671:string)  [unwired: 1 in]
              n262 = To Upper Case(1:w671) -> (0:w670:string)
              n263 = Not Equal?(x=w670, y=w669) -> (x != y?=w667:bool)
              n264 = Compound Arithmetic op=OR(invert w667, w666) -> (w665:bool)
            }
            n265 = Or(x=w663, y=w656) -> (x .or. y?=w657:bool)
            n266 = in-place-cluster #14("skvc"=w659) -> (w653:cluster{"skvc":string[][]})
          }
          n267 = in-place-array #12(w651) -> (w641:bool[])  [unwired: 1 out]
          n268 = in-place-array #13(w653) -> (w644:cluster{"skvc":string[][]}[])  [unwired: 1 out]
        }
        n269 = Bundle By Name(cluster=w648, "Modified"=w641, "Files"=w644, "Found"=w640, "skvc"=string[] []) -> (w647:T2)
      }
    }
    n270 = Empty Array?(array=w18) -> (empty?=w17:bool)
  }
  "error out" <- w11
  n271 = disable-structure shown="Disabled" {
    frame Disabled {
      n272 = Empty String/Path?() -> (string/path=w676:string, empty?=w675:bool)
      n273 = case "Empty?" shown="True" w675 {
        tunnel: _ -> [w686 w689]
        tunnel: [w686 w688] -> w673
        frame False {
        }
        frame True {
          n274 = xnode "Error Ring"() -> ("error out"=w687:errorcluster)
          n275 = Merge Errors(w689, w687) -> (w688:errorcluster)
        }
      }
      n276 = Empty String/Path?() -> (string/path=w672:string, empty?=w674:bool)
      n277 = case "Empty?" shown="True" w674 {
        tunnel: w673 -> [w677 w680]
        tunnel: [w677 w679] -> _
        frame False {
        }
        frame True {
          n278 = xnode "Error Ring"() -> ("error out"=w678:errorcluster)
          n279 = Merge Errors(w680, w678) -> (w679:errorcluster)
        }
      }
    }
    frame Enabled {
    }
  }
  n280 = Unbundle By Name(w3) -> ("Found"=→"Found?":bool, "skvc"=→"skvc out":string[])
  "INI Path out" <- "INI Path in"
